vi "Bind Multiple Terminal Values.vi"(4 "Ignore Past Updates? (F)":bool, 6 "Value Changes Only? (T)":bool=TRUE, 8 "error in (no error)":errorcluster, 10 "Ctl Refnums":refnum<vi>[](array[refnum]), 11 "IViewable in":refnum<class "IViewable.lvclass">) -> (0 "error out":errorcluster, 3 "IViewable out":refnum<class "IViewable.lvclass">)   [LabVIEW 2020, in "MVA Framework.lvlib" / "IViewable.lvlib" / "IViewable.lvclass"]
doc: "将多个控制终端值（控件或指示器）绑定到已发布的数据，其名称和类型与有线终端引用的名称和类型匹配。"
uses:
  IViewable.lvclass
  IViewable.lvclass/IViewable.ctl
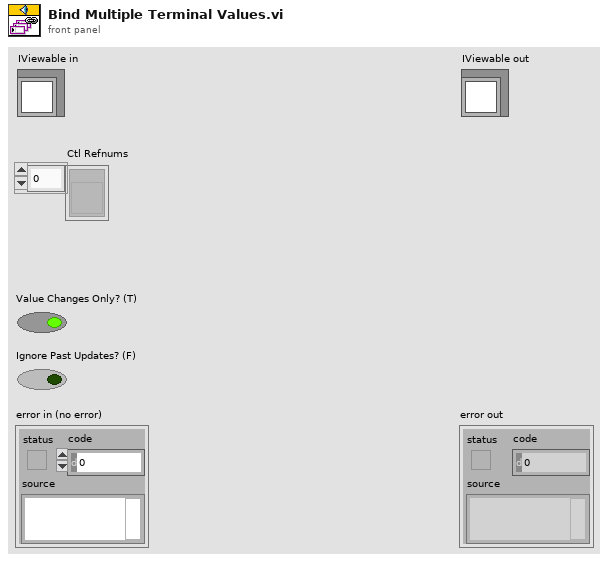
[diagram p1: front panel]
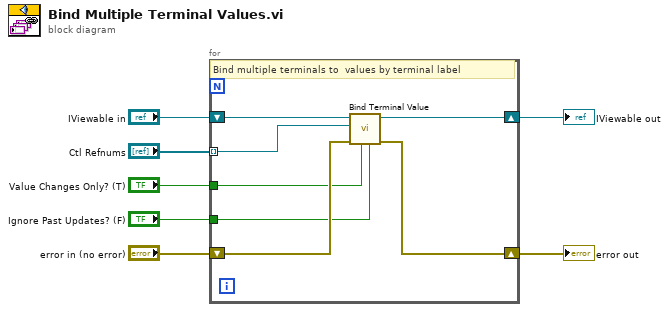
[diagram p0: block diagram]
diagram:
  n1 = for {
    shift-right: [w13] -> w6
    shift-left: "IViewable in" -> [w14]
    shift-right: [w11] -> w4
    shift-left: "error in (no error)" -> [w12]
    tunnel: "Ctl Refnums" -> [w10] mode=indexing
    tunnel: "Value Changes Only? (T)" -> [w9]
    tunnel: "Ignore Past Updates? (F)" -> [w8]
    # "Bind multiple terminals to  values by terminal label"
    n2 = call "Bind Terminal Value.vi"("Ignore Past Updates? (F)"=w8, "Value Changes Only? (T)"=w9, "error in (no error)"=w12, "Ctl Refnum"=w10, "IViewable in"=w14) -> ("error out"=w11:errorcluster, "IViewable out"=w13:refnum<class "IViewable.lvclass">)  [unwired: 5 in]
  }
  "error out" <- w4
  "IViewable out" <- w6
